vi "Autonomous Independent.vi"   [LabVIEW 2016]
doc: "This VI is called when autonomous begins, and will automatically be terminated when autonomous ends. You can carry out timed or sensor driven robot movement independently without needing to return to the caller."
uses:
  <vilib>/Rock Robotics/Network Tables/NT Read Number.vi
  <vilib>/Rock Robotics/Network Tables/NT Read Boolean.vi
  Robot Global Data.vi
panel:
  # "Be sure to right-click and choose Data Operations>>Make Current Value default if you want to save the array values with the VI"
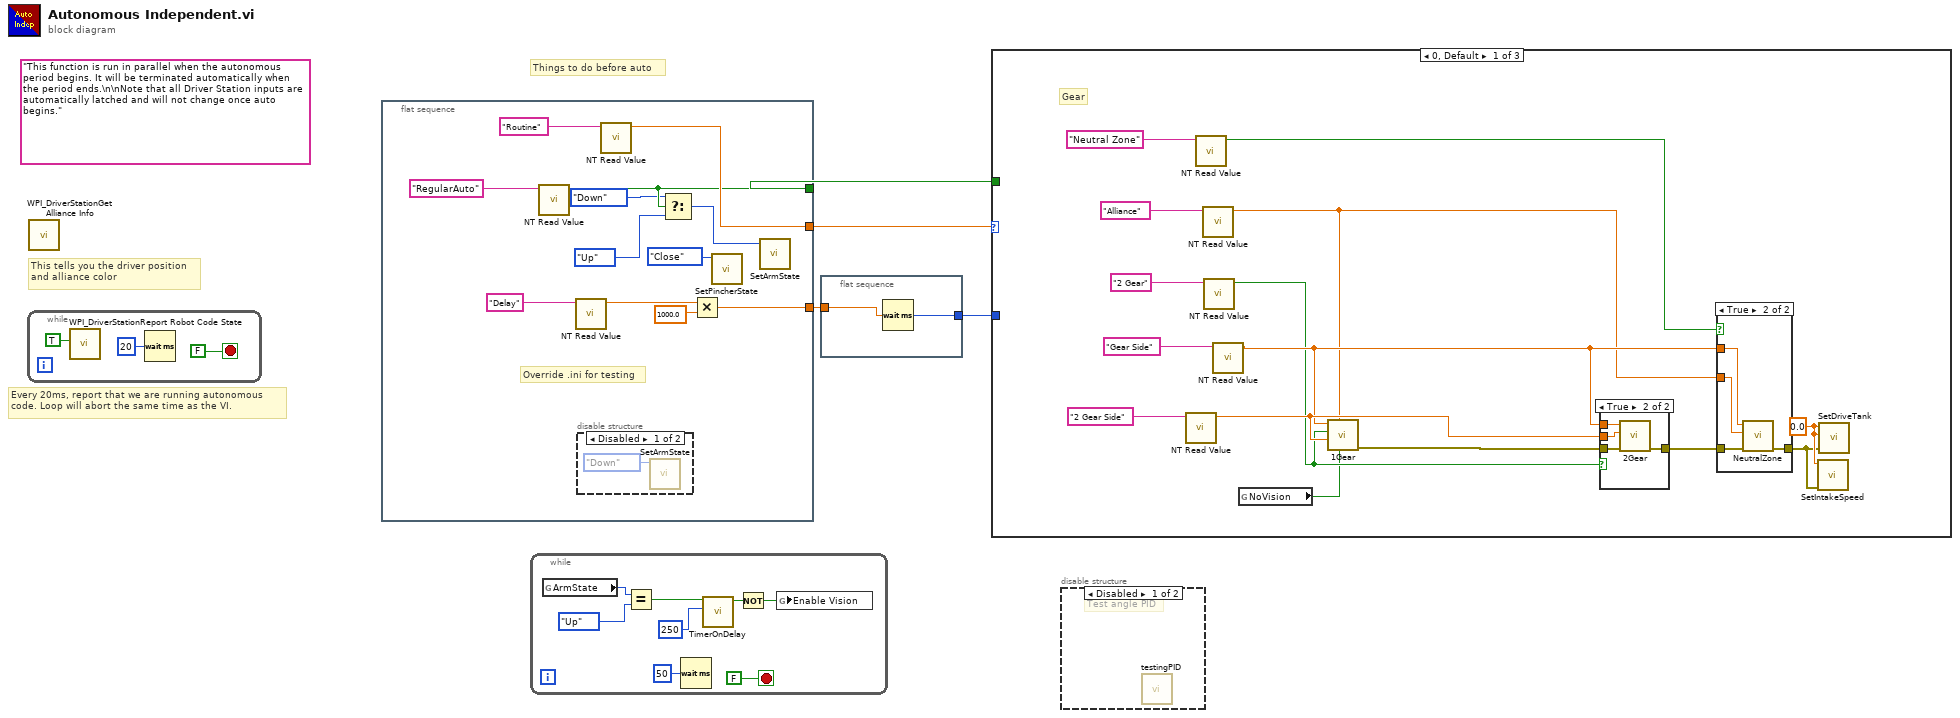
[diagram p0: block diagram]
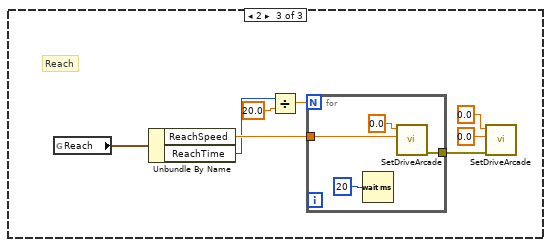
[diagram p5: hidden frame]
diagram:
  (unwired) "This function is run in parallel when the autonomous period begins. It will be terminated automatically when the period ends.\n\nNote that all Driver Station inputs are automatically latched and will not change once auto begins."
  # "Things to do before auto"
  # "Every 20ms, report that we are running autonomous\ncode. Loop will abort the same time as the VI."
  # "This tells you the driver position\nand alliance color"
  n1 = while {
    stop <- FALSE stop-if-true
    n2 = call <vilib>:"WPI_DriverStationReport Robot Code State.vi"("Autonomous"=TRUE) -> ()  [unwired: 10 in, 1 out]
    n3 = Wait (ms)(milliseconds to wait=u32 20) -> ()  [unwired: 1 out]
  }
  n4 = call <vilib>:"WPI_DriverStationGet Alliance Info.vi"() -> ()  [unwired: 12 out]
  n5 = flat-sequence {
    tunnel: [w17] -> w4
    tunnel: [w13] -> w3
    tunnel: [w11] -> w1
    frame #0 {
      # "Override .ini for testing"
      n6 = call-poly <vilib>:"NT Read Value.vi"("Name"="RegularAuto") -> ("Boolean"=w11:bool)  [unwired: 9 in, 1 out]
      n7 = call-poly <vilib>:"NT Read Value.vi"("Name"="Delay") -> ("Numeric"=w15:dbl)  [unwired: 9 in, 1 out]
      n8 = disable-structure shown="Disabled" {
        frame Disabled {
          n9 = call "SetArmState.vi"("ArmState"=enum16{"Up", "Down"}."Down") -> ()  [unwired: 10 in, 1 out]
        }
        frame Enabled {
        }
      }
      n10 = call-poly <vilib>:"NT Read Value.vi"("Name"="Routine") -> ("Numeric"=w17:dbl)  [unwired: 9 in, 1 out]
      n11 = Select(t=enum16{"Up", "Down"}."Down" ("ArmState"), s=w11, f=enum16{"Up", "Down"}."Up" ("ArmState")) -> (s? t:f=w10:enum16{"Up", "Down"})
      n12 = Multiply(x=w15, y=1000.0) -> (x*y=w13:dbl)
      n13 = call "SetPincherState.vi"("PincherState"=enum16{"Open", "Close"}."Close") -> ()  [unwired: 10 in, 1 out]
      n14 = call "SetArmState.vi"("ArmState"=w10) -> ()  [unwired: 10 in, 1 out]
    }
  }
  n15 = while {
    stop <- FALSE stop-if-true
    n16 = global read "Robot Global Data.vi" "ArmState"() -> (w26:enum16{"Up", "Down"})
    n17 = Equal?(x=w26, y=enum16{"Up", "Down"}."Up") -> (x = y?=w22:bool)
    n18 = Wait (ms)(milliseconds to wait=u32 50) -> ()  [unwired: 1 out]
    n19 = call "TimerOnDelay.vi"("Time Limit"=u32 250, "Input"=w22) -> ("Output"=w23:bool)  [unwired: 9 in]
    n20 = Not(x=w23) -> (.not. x?=w21:bool)
    n21 = global write "Robot Global Data.vi" "Enable Vision"(w21) -> ()
  }
  n22 = flat-sequence {
    tunnel: w3 -> [w30]
    tunnel: [w29] -> w2
    frame #0 {
      n23 = Wait (ms)(milliseconds to wait=w30) -> (millisecond timer value=w29:u32)
    }
  }
  n24 = case shown="0, Default" w4 {
    tunnel: w2 -> [_ _ _]
    tunnel: w1 -> [_ _ _]
    frame 0, Default {
      w44 = 0.0 ("Left")
      # "Gear"
      n25 = call-poly <vilib>:"NT Read Value.vi"("Name"="2 Gear Side") -> ("Numeric"=w37:dbl)  [unwired: 9 in, 1 out]
      n26 = call-poly <vilib>:"NT Read Value.vi"("Name"="Neutral Zone") -> ("Boolean"=w34:bool)  [unwired: 9 in, 1 out]
      n27 = call-poly <vilib>:"NT Read Value.vi"("Name"="Alliance") -> ("Numeric"=w31:dbl)  [unwired: 9 in, 1 out]
      n28 = call-poly <vilib>:"NT Read Value.vi"("Name"="2 Gear") -> ("Boolean"=w35:bool)  [unwired: 9 in, 1 out]
      n29 = call-poly <vilib>:"NT Read Value.vi"("Name"="Gear Side") -> ("Numeric"=w36:dbl)  [unwired: 9 in, 1 out]
      n30 = global read "Robot Global Data.vi" "NoVision"() -> (w33:bool)
      n31 = call "1Gear.vi"("No Vision"=w33, "Alliance"=w31, "2 Gear Side"=w37, "2 Gear"=w35, "Gear Side"=w36) -> ("error out"=w32:errorcluster)  [unwired: 6 in]
      n32 = case shown="True" w35 {
        tunnel: w36 -> [_ w55]
        tunnel: w37 -> [_ w54]
        tunnel: w32 -> [w51 w53]
        tunnel: [w51 w52] -> w45
        frame False {
        }
        frame True {
          n33 = call "2Gear.vi"("error in"=w53, "2 Gear Side"=w54, "Gear Side"=w55) -> ("error out"=w52:errorcluster)  [unwired: 8 in]
        }
      }
      n34 = case shown="True" w34 {
        tunnel: w45 -> [w46 w49]
        tunnel: [w46 w50] -> w43
        tunnel: w31 -> [_ w48]
        tunnel: w36 -> [_ w47]
        frame False {
        }
        frame True {
          n35 = call "NeutralZone.vi"("error in"=w49, "Alliance"=w48, "Gear Side"=w47) -> ("error out"=w50:errorcluster)  [unwired: 8 in]
        }
      }
      n36 = call "SetIntakeSpeed.vi"("error in"=w43, "Speed"=w44) -> ()  [unwired: 9 in, 1 out]
      n37 = call "SetDriveTank.vi"("error in"=w43, "Right"=w44, "Left"=w44) -> ()  [unwired: 8 in, 1 out]
    }
    frame 1 {
      # "Do nothing"
      # "Except maybe lower arm or outtake gear"
    }
    frame 2 {
      # "Reach"
      n38 = global read "Robot Global Data.vi" "Reach"() -> (w62:cluster{"ReachSpeed":dbl, "ReachTime":u32})
      n39 = Unbundle By Name(w62) -> ("ReachSpeed"=w63:dbl, "ReachTime"=w60:u32)
      n40 = Divide(x=w60, y=20.0) -> (x/y=w61:dbl)
      n41 = for {
        N: w61 -> [_]
        tunnel: w63 -> [w67]
        tunnel: [w64] -> w56
        n42 = Wait (ms)(milliseconds to wait=u32 20) -> ()  [unwired: 1 out]
        n43 = call "SetDriveArcade.vi"("Forward"=w67, "Turn"=0.0) -> ("error out"=w64:errorcluster)  [unwired: 9 in]
      }
      n44 = call "SetDriveArcade.vi"("error in"=w56, "Forward"=0.0, "Turn"=0.0 ("Forward")) -> ()  [unwired: 8 in, 1 out]
    }
  }
  n45 = disable-structure shown="Disabled" {
    frame Disabled {
      # "Test angle PID"
      n46 = call "testingPID.vi"() -> ()  [unwired: 12 in]
    }
    frame Enabled {
    }
  }
